vi "VI Tree.vi"   [LabVIEW 2018, in "Agilent MXA Series.lvlib"]
doc: "This is the instrument driver for Agilent-Keysight MXA,EXA,PXA and CXA Series. The VI Tree displays all the user-callable VIs of the instrument driver in an organized table."
uses:
  Agilent MXA Series.lvlib
  Configure/Configure Frequency (Start Stop).vi
  Configure/Marker/Configure Marker Trace (Swept SA).vi
  Configure/Marker/Configure Marker Type (Swept SA).vi
  Configure/Configure Level (Normal).vi
  Data/Read Trace (Swept SA).vi
  Data/Low Level/Fetch Trace (Swept SA).vi
  Data/Read Measurement (Swept SA).vi
  Data/Low Level/Fetch Measurement (Swept SA).vi
  Configure/Trigger/Configure Trigger (Normal).vi
  Configure/Measurement/Configure Range Table (Spurious Emissions - IF Gain).vi
  Configure/Measurement/Configure Offset and Limits (Adjacent Channel Power - VBW and RBW).vi
  Configure/Measurement/Configure Carrier (Carrier Count).vi
  Configure/Configure IF Gain (Swept SA).vi
  Configure/Measurement/Configure Measurement (Spectrum Emissions Mask).vi
  Configure/Measurement/Configure Reference Channel (Others).vi
panel:
  # "(c) 2007-2015 National Instruments.  ALL RIGHTS RESERVED."
  # "SEE DIAGRAM\nFOR VI TREE."
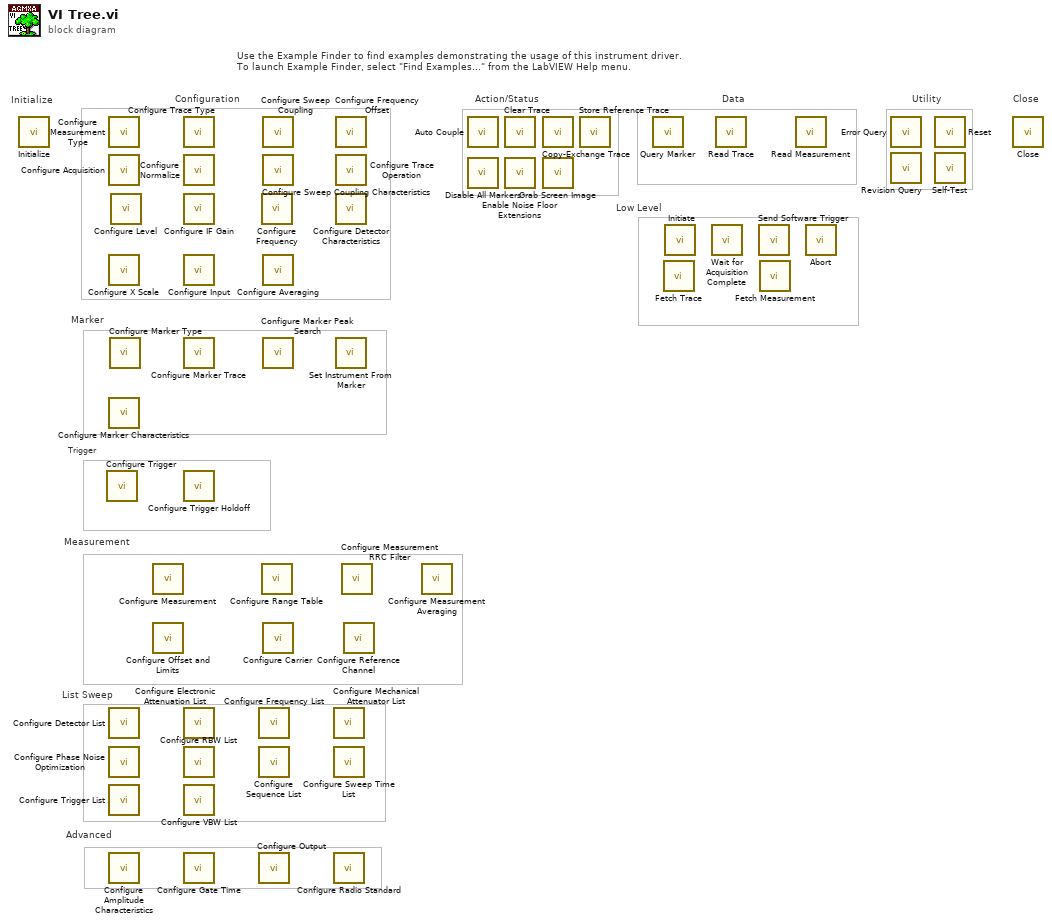
[diagram p0: block diagram]
diagram:
  # "Low Level"
  # "List Sweep"
  # "Trigger"
  # "Measurement"
  # "Marker"
  # "Advanced"
  # "Use the Example Finder to find examples demonstrating the usage of this instrument driver.\nTo launch Example Finder, select \"Find Examples...\" from the LabVIEW Help menu."
  # "Configuration"
  # "Utility"
  # "Data"
  # "Action/Status"
  # "Close"
  # "Initialize"
  n1 = call "Initialize.vi"() -> ()  [unwired: 10 in, 2 out]
  n2 = call-poly "Configure Trigger.vi"() -> ()  [unwired: 14 in, 2 out]
  n3 = call "Configure Measurement Type.vi"() -> ()  [unwired: 10 in, 2 out]
  n4 = call "Configure Acquisition.vi"() -> ()  [unwired: 14 in, 2 out]
  n5 = call "Configure X Scale.vi"() -> ()  [unwired: 10 in, 2 out]
  n6 = call "Configure Marker Characteristics.vi"() -> ()  [unwired: 10 in, 2 out]
  n7 = call "Configure Detector List.vi"() -> ()  [unwired: 10 in, 2 out]
  n8 = call "Configure Phase Noise Optimization.vi"() -> ()  [unwired: 10 in, 2 out]
  n9 = call "Configure Trigger List.vi"() -> ()  [unwired: 14 in, 2 out]
  n10 = call "Configure Amplitude Characteristics.vi"() -> ()  [unwired: 14 in, 2 out]
  n11 = call-poly "Configure Marker Type.vi"() -> ()  [unwired: 14 in, 2 out]
  n12 = call-poly "Configure Level.vi"() -> ()  [unwired: 14 in, 2 out]
  n13 = call-poly "Configure Measurement.vi"() -> ()  [unwired: 14 in, 2 out]
  n14 = call-poly "Configure Offset and Limits.vi"() -> ()  [unwired: 14 in, 2 out]
  n15 = call "Configure Trace Type.vi"() -> ()  [unwired: 10 in, 2 out]
  n16 = call "Configure Normalize.vi"() -> ()  [unwired: 10 in, 2 out]
  n17 = call-poly "Configure IF Gain.vi"() -> ()  [unwired: 10 in, 2 out]
  n18 = call "Configure Input.vi"() -> ()  [unwired: 14 in, 2 out]
  n19 = call-poly "Configure Marker Trace.vi"() -> ()  [unwired: 10 in, 2 out]
  n20 = call "Configure Trigger Holdoff.vi"() -> ()  [unwired: 10 in, 2 out]
  n21 = call "Configure Electronic Attenuation List.vi"() -> ()  [unwired: 10 in, 2 out]
  n22 = call "Configure RBW List.vi"() -> ()  [unwired: 10 in, 2 out]
  n23 = call "Configure VBW List.vi"() -> ()  [unwired: 10 in, 2 out]
  n24 = call "Configure Gate Time.vi"() -> ()  [unwired: 14 in, 2 out]
  n25 = call "Configure Frequency List.vi"() -> ()  [unwired: 10 in, 2 out]
  n26 = call "Configure Sequence List.vi"() -> ()  [unwired: 10 in, 2 out]
  n27 = call "Configure Output.vi"() -> ()  [unwired: 10 in, 2 out]
  n28 = call-poly "Configure Frequency.vi"() -> ()  [unwired: 10 in, 2 out]
  n29 = call-poly "Configure Range Table.vi"() -> ()  [unwired: 14 in, 2 out]
  n30 = call "Configure Sweep Coupling.vi"() -> ()  [unwired: 14 in, 2 out]
  n31 = call "Configure Sweep Coupling Characteristics.vi"() -> ()  [unwired: 14 in, 2 out]
  n32 = call "Configure Averaging.vi"() -> ()  [unwired: 10 in, 2 out]
  n33 = call "Configure Marker Peak Search.vi"() -> ()  [unwired: 14 in, 2 out]
  n34 = call-poly "Configure Carrier.vi"() -> ()  [unwired: 14 in, 2 out]
  n35 = call "Configure Mechanical Attenuator List.vi"() -> ()  [unwired: 10 in, 2 out]
  n36 = call "Configure Sweep Time List.vi"() -> ()  [unwired: 10 in, 2 out]
  n37 = call "Configure Radio Standard.vi"() -> ()  [unwired: 14 in, 2 out]
  n38 = call "Configure Frequency Offset.vi"() -> ()  [unwired: 10 in, 2 out]
  n39 = call "Configure Trace Operation.vi"() -> ()  [unwired: 14 in, 2 out]
  n40 = call "Configure Detector Characteristics.vi"() -> ()  [unwired: 10 in, 2 out]
  n41 = call "Set Instrument From Marker.vi"() -> ()  [unwired: 10 in, 2 out]
  n42 = call "Configure Measurement RRC Filter.vi"() -> ()  [unwired: 10 in, 2 out]
  n43 = call-poly "Configure Reference Channel.vi"() -> ()  [unwired: 14 in, 2 out]
  n44 = call "Configure Measurement Averaging.vi"() -> ()  [unwired: 10 in, 2 out]
  n45 = call "Auto Couple.vi"() -> ()  [unwired: 10 in, 2 out]
  n46 = call "Disable All Markers.vi"() -> ()  [unwired: 10 in, 2 out]
  n47 = call "Clear Trace.vi"() -> ()  [unwired: 10 in, 2 out]
  n48 = call "Enable Noise Floor Extensions.vi"() -> ()  [unwired: 10 in, 2 out]
  n49 = call "Copy-Exchange Trace.vi"() -> ()  [unwired: 10 in, 2 out]
  n50 = call "Grab Screen Image.vi"() -> ()  [unwired: 10 in, 2 out]
  n51 = call "Store Reference Trace.vi"() -> ()  [unwired: 10 in, 2 out]
  n52 = call "Query Marker.vi"() -> ()  [unwired: 8 in, 4 out]
  n53 = call-poly "Fetch Trace.vi"() -> ()  [unwired: 12 in, 4 out]
  n54 = call "Initiate.vi"() -> ()  [unwired: 10 in, 2 out]
  n55 = call "Wait for Acquisition Complete.vi"() -> ()  [unwired: 10 in, 2 out]
  n56 = call-poly "Read Trace.vi"() -> ()  [unwired: 9 in, 3 out]
  n57 = call "Send Software Trigger.vi"() -> ()  [unwired: 10 in, 2 out]
  n58 = call-poly "Fetch Measurement.vi"() -> ()  [unwired: 13 in, 3 out]
  n59 = call-poly "Read Measurement.vi"() -> ()  [unwired: 13 in, 3 out]
  n60 = call "Abort.vi"() -> ()  [unwired: 10 in, 2 out]
  n61 = call "Error Query.vi"() -> ()  [unwired: 8 in, 4 out]
  n62 = call "Revision Query.vi"() -> ()  [unwired: 8 in, 4 out]
  n63 = call "Reset.vi"() -> ()  [unwired: 10 in, 2 out]
  n64 = call "Self-Test.vi"() -> ()  [unwired: 8 in, 4 out]
  n65 = call "Close.vi"() -> ()  [unwired: 11 in, 1 out]
